vi "Visualize FFT.vi"(6 "Frequency Metedata":T2, 8 "error in (no error)":errorcluster, 9 "Signal Density Plot":T3, 10 "FFT Data":T1, 11 "Application Manager in":refnum<class "Application Manager.lvclass">) -> (0 "error out":errorcluster, 3 "Application Manager out":refnum<class "Application Manager.lvclass">)   [LabVIEW 2020, in "Application Manager.lvlib" / "Application Manager.lvclass"]
uses:
  Application Manager.lvclass
  UI/UI Root/UI Root/Signal Density Plot Data.ctl
  <vilib>/Utility/miscctls.llb/LVOffsetAndMultiplierTypeDef.ctl
  UI/UI Root/UI Root/Frequency Metadata.ctl
  UI/UI Root/UI Root/FFT Plot Data.ctl
  Application Manager.lvclass/Application Manager.ctl
  UI/UI Root/UI Root Messages/Visualise FFT Msg/Visualise FFT Msg.lvclass/Visualise FFT Msg.ctl
  <vilib>/ActorFramework/Message Enqueuer/Message Enqueuer.lvclass/Message Enqueuer.ctl
  <vilib>/ActorFramework/Message Enqueuer/Enqueue.vi
  UI/UI Root/UI Root Messages/Visualise FFT Msg/Visualise FFT Msg.lvclass
  C:/Program Files/National Instruments/LabVIEW 2025/vi.lib/ActorFramework/Message/Message.lvclass
  <vilib>/ActorFramework/Message Priority Queue/Priority Enqueue.vi
  UI/UI Root/UI Root/UI Root.lvclass
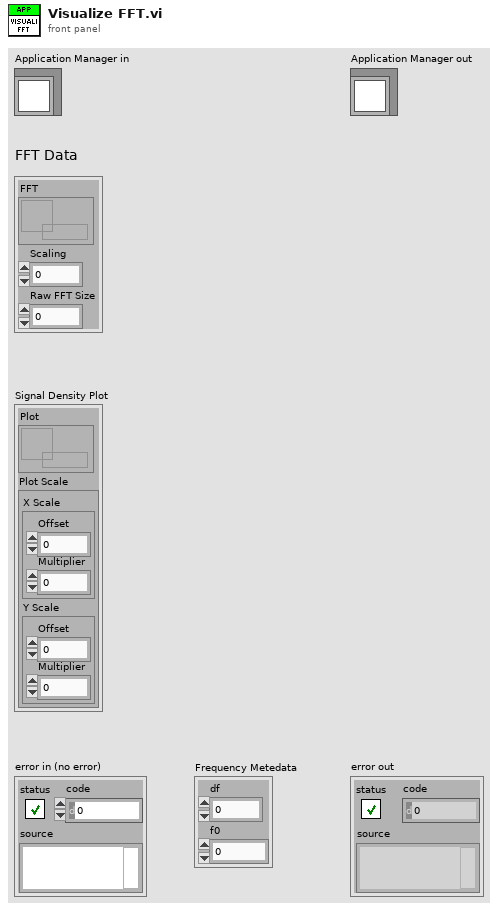
[diagram p1: front panel]
types:
  T1 = typedef "UI Root.lvlib/UI Root.lvclass/FFT Plot Data.ctl" = cluster{"FFT":refnum<data-value>, "Scaling":dbl, "Raw FFT Size":i32}
  T2 = typedef "UI Root.lvlib/UI Root.lvclass/Frequency Metadata.ctl" = cluster{"df":dbl, "f0":dbl}
  T3 = typedef "UI Root.lvlib/UI Root.lvclass/Signal Density Plot Data.ctl" = cluster{"Plot":refnum<data-value>, "Plot Scale":cluster{"X Scale":T4, "Y Scale":T4}}
  T4 = typedef "LVOffsetAndMultiplierTypeDef.ctl" = cluster{"Offset":dbl, "Multiplier":dbl}
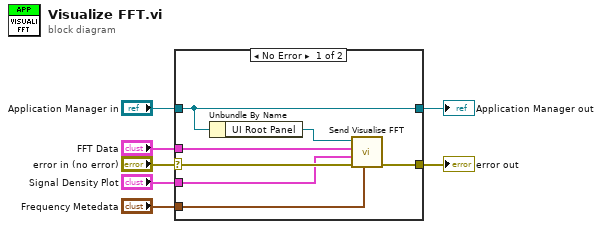
[diagram p0: block diagram]
diagram:
  n1 = case shown="No Error" "error in (no error)" {
    selector: "error in (no error)" -> [w11 w16]
    tunnel: [w10 w16] -> w6
    tunnel: [w14 w15] -> w4
    tunnel: "Application Manager in" -> [w14 w15]
    tunnel: "FFT Data" -> [w12 _]
    tunnel: "Signal Density Plot" -> [w9 _]
    tunnel: "Frequency Metedata" -> [w8 _]
    frame No Error {
      n2 = Unbundle By Name(w14) -> ("UI Root Panel"=w13:refnum<class "Message Enqueuer.lvclass">)
      n3 = call "Send Visualise FFT.vi"("Frequency Metedata"=w8, "error in (no error)"=w11, "Signal Density Plot"=w9, "FFT Data"=w12, "Message Enqueuer"=w13) -> ("error out"=w10:errorcluster)  [unwired: 5 in, 1 out]
    }
    frame Error {
    }
  }
  "error out" <- w6
  "Application Manager out" <- w4
